vi "LabVIEW SSH via PuTTY plink.vi"() -> ()   [LabVIEW 2020]
panel:
  in  "Hide DOS\nWindow?":bool
  out "Command Executed":string
  out "Errors":string
  in  "Password":string="password"
  in  "Host":string="host.domain.com"
  in  "Username":string="username"
  in  "Command(s) to Execute":string="pwd"
  out "Command Return Value(s)":string
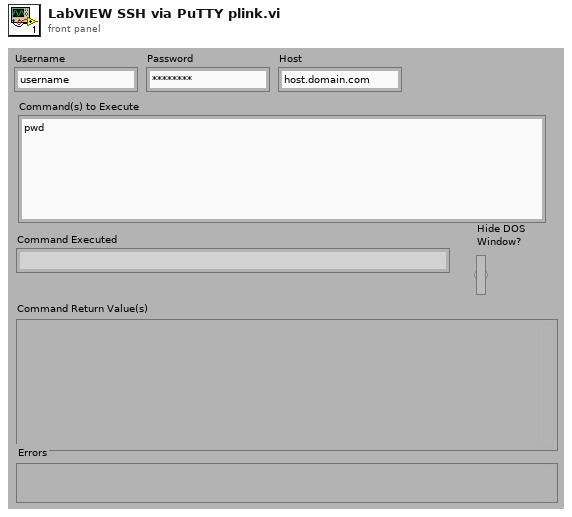
[diagram p1: front panel]
types:
  T1 = enum16{"open", "replace", "create", "open or create", "replace or create", "replace or create with confirmation"}
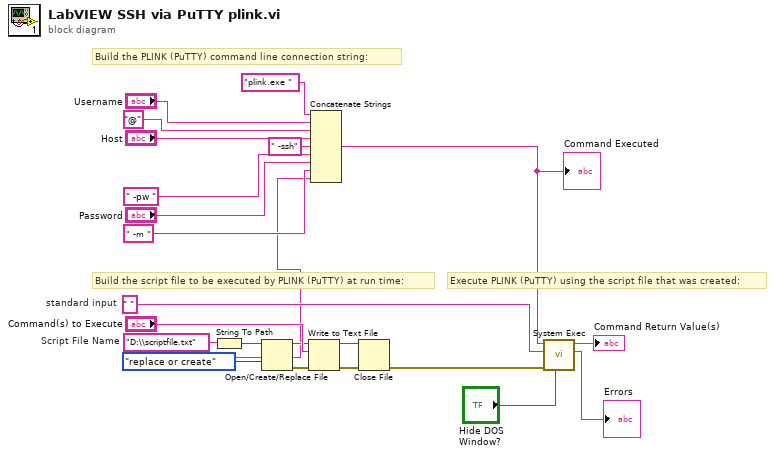
[diagram p0: block diagram]
diagram:
  w14 = " "  # standard input
  w2 = "D:\\scriptfile.txt"  # Script File Name
  # "Execute PLINK (PuTTY) using the script file that was created:"
  # "Build the script file to be executed by PLINK (PuTTY) at run time:"
  # "Build the PLINK (PuTTY) command line connection string:"
  n1 = String To Path(string=w2) -> (path=w6:path)
  n2 = Open/Create/Replace File(file path (use dialog)=w6, operation (0:open)=T1."replace or create") -> (refnum out=w17:refnum<file>, error out=w16:errorcluster)  [unwired: 4 in, 1 out]
  n3 = Write to Text File(file (use dialog)=w17, text="Command(s) to Execute", error in=w16) -> (refnum out=w20:refnum<file>, error out=w19:errorcluster)  [unwired: 2 out]
  n4 = Concatenate Strings("plink.exe " ("command line"), "Username", "@" ("string"), "Host", " -ssh" ("string"), " -pw " ("string"), "Password", " -m " ("string"), w2) -> (w7:string)
  "Command Executed" <- w7
  n5 = Close File(refnum=w20, error in=w19) -> (error out=w18:errorcluster)  [unwired: 1 out]
  n6 = call <vilib>:"System Exec.vi"("run minimized? (F)"="Hide DOS\nWindow?", "error in (no error)"=w18, "standard input"=w14, "command line"=w7) -> ("standard error"=→"Errors":string, "standard output"=→"Command Return Value(s)":string)  [unwired: 2 in, 4 out]
